vi "VIP_Post-Install Custom Action.vi"(10 "Variant":variant) -> (0 "error out":errorcluster)   [LabVIEW 2021]
uses:
  <vilib>/Utility/sysdir.llb/System Directory Type.ctl
  <userlib>/_OpenG.lib/lvzip/fileutil.llb/subVIs/FILE Rename (Path)__ogtk.vi
  <userlib>/_OpenG.lib/file/file.llb/openg_file.lvlib
  <userlib>/_OpenG.lib/file/file.llb/Convert File Extension (Path)__ogtk.vi
panel:
  # "POST INSTALL"
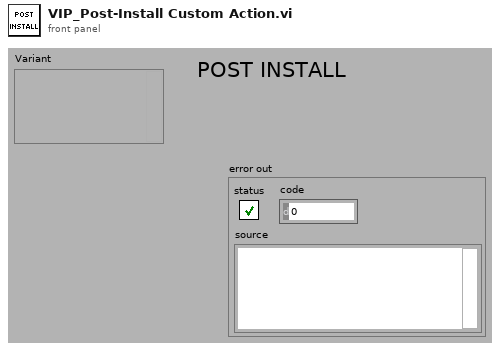
[diagram p1: front panel]
types:
  T1 = typedef "System Directory Type.ctl" = i32
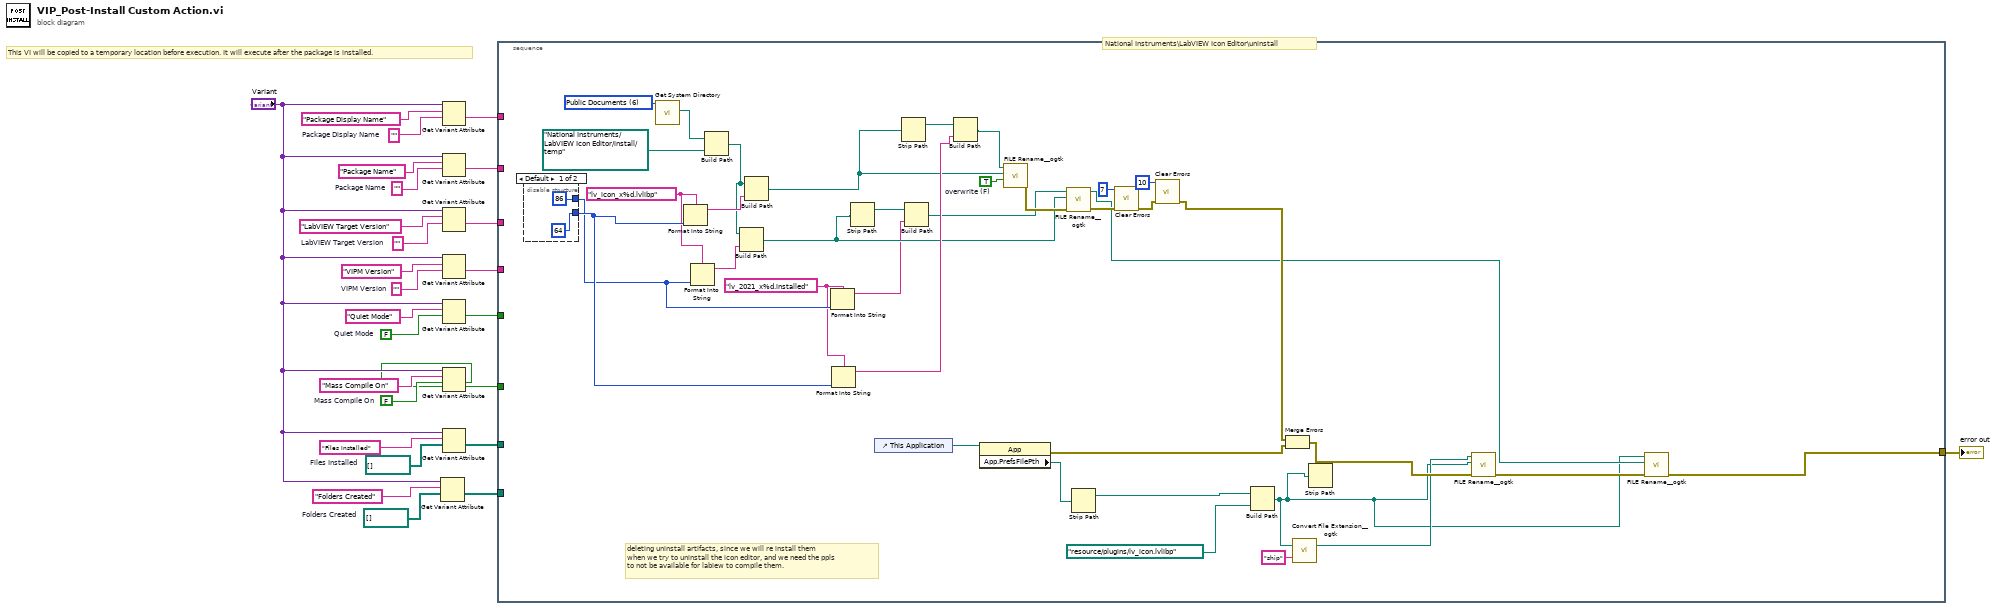
[diagram p0: block diagram]
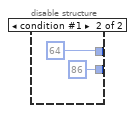
[diagram p2: hidden frame]
diagram:
  w10 = path[] []  # Folders Created
  w11 = path[] []  # Files Installed
  w15 = FALSE  # Mass Compile On
  w16 = ""  # Package Display Name
  w17 = FALSE  # Quiet Mode
  w20 = ""  # VIPM Version
  w22 = ""  # LabVIEW Target Version
  w24 = ""  # Package Name
  # "National Instruments\\LabVIEW Icon Editor\\uninstall"
  # "This VI will be copied to a temporary location before execution. It will execute after the package is installed."
  n1 = Get Variant Attribute(Variant="Variant", name="Folders Created", default value (empty Variant)=w10) -> (value=w2:path[])  [unwired: 1 in, 3 out]
  n2 = Get Variant Attribute(Variant="Variant", name="Package Display Name", default value (empty Variant)=w16) -> (value=w9:string)  [unwired: 1 in, 3 out]
  n3 = Get Variant Attribute(Variant="Variant", name="Package Name", default value (empty Variant)=w24) -> (value=w8:string)  [unwired: 1 in, 3 out]
  n4 = Get Variant Attribute(Variant="Variant", name="LabVIEW Target Version", default value (empty Variant)=w22) -> (value=w7:string)  [unwired: 1 in, 3 out]
  n5 = Get Variant Attribute(Variant="Variant", name="VIPM Version", default value (empty Variant)=w20) -> (value=w6:string)  [unwired: 1 in, 3 out]
  n6 = Get Variant Attribute(Variant="Variant", name="Quiet Mode", default value (empty Variant)=w17) -> (value=w3:bool)  [unwired: 1 in, 3 out]
  n7 = Get Variant Attribute(Variant="Variant", name="Mass Compile On", default value (empty Variant)=w15) -> (value=w5:bool)  [unwired: 1 in, 3 out]
  n8 = Get Variant Attribute(Variant="Variant", name="Files Installed", default value (empty Variant)=w11) -> (value=w4:path[])  [unwired: 1 in, 3 out]
  n9 = stacked-sequence {
    tunnel: [w28] -> w1
    tunnel: w9 -> [_]
    tunnel: w8 -> [_]
    tunnel: w7 -> [_]
    tunnel: w6 -> [_]
    tunnel: w5 -> [_]
    tunnel: w4 -> [_]
    tunnel: w3 -> [_]
    tunnel: w2 -> [_]
    frame #0 {
      w41 = "lv_2021_x%d.installed" ("format string")
      w58 = TRUE  # overwrite (F)
      w40 = "lv_icon_x%d.lvlibp" ("format string")
      w63 = T1 6 items=["User Home"=0, "User Desktop"=1, "User Documents"=2, "User Application Data"=3, "User Preferences"=4, "User Temporary"=5, "Public Documents"=6, "Public Application Data"=7, "Public Preferences"=8, "Public Cache"=13, "System Core Libraries"=9, "System Installed Libraries"=10, "Application Files"=11, "Boot Volume Root"=12] ("system directory type")
      # "deleting uninstall artifacts, since we will re install them\nwhen we try to uninstall the icon editor, and we need the ppls\nto not be available for labiew to compile them."
      n10 = disable-structure shown="Default" {
        disable-tunnel: [64 ("code") 86 ("code")] -> w57
        disable-tunnel: [86 ("code") 64 ("code")] -> w46
        frame condition #0 (active) {
        }
        frame condition #1 {
        }
      }
      n11 = call <vilib>:"Get System Directory.vi"("system directory type"=w63) -> ("system directory"=w35:path)  [unwired: 10 in]
      n12 = Format Into String(format string=w40, w57) -> (resulting string=w55:string)  [unwired: 2 in, 1 out]
      n13 = Format Into String(format string=w40, w46) -> (resulting string=w50:string)  [unwired: 2 in, 1 out]
      n14 = Build Path(base path=w35, name or relative path=path "National Instruments/LabVIEW Icon Editor/install/temp" ("source path")) -> (appended path=w51:path)
      n15 = Build Path(base path=w51, name or relative path=w50) -> (appended path=w47:path)
      n16 = Build Path(base path=w51, name or relative path=w55) -> (appended path=w36:path)
      n17 = Format Into String(format string=w41, w46) -> (resulting string=w45:string)  [unwired: 2 in, 1 out]
      n18 = Format Into String(format string=w41, w57) -> (resulting string=w53:string)  [unwired: 2 in, 1 out]
      n19 = Strip Path(path=w47) -> (stripped path=w48:path)  [unwired: 1 out]
      n20 = control-ref of="This Application"() -> (w62:refnum<vi>)
      n21 = Strip Path(path=w36) -> (stripped path=w54:path)  [unwired: 1 out]
      n22 = Build Path(base path=w48, name or relative path=w45) -> (appended path=w44:path)
      n23 = Build Path(base path=w54, name or relative path=w53) -> (appended path=w52:path)
      n24 = property class="App"(reference=w62) -> (error out=w59:errorcluster, "App.PrefsFilePth"=w60:path)  [unwired: 1 in, 1 out]
      n25 = call-poly <userlib>:"FILE Rename__ogtk.vi"("overwrite (F)"=w58, "source path"=w36, "target path"=w52) -> ("error out"=w49:errorcluster)  [unwired: 7 in, 1 out]
      n26 = call-poly <userlib>:"FILE Rename__ogtk.vi"("error in (no error)"=w49, "source path"=w47, "target path"=w44) -> ("error out"=w43:errorcluster, "dup target path"=w30:path)  [unwired: 7 in]
      n27 = Strip Path(path=w60) -> (stripped path=w33:path)  [unwired: 1 out]
      n28 = call <vilib>:"Clear Errors.vi"("error in (no error)"=w43, "specific error code to clear (0: all)"=7) -> ("error out"=w39:errorcluster)  [unwired: 4 in, 1 out]
      n29 = call <vilib>:"Clear Errors.vi"("error in (no error)"=w39, "specific error code to clear (0: all)"=10) -> ("error out"=w38:errorcluster)  [unwired: 4 in, 1 out]
      n30 = Build Path(base path=w33, name or relative path=path "resource/plugins/lv_icon.lvlibp") -> (appended path=w27:path)
      n31 = Merge Errors(w38, w59) -> (w32:errorcluster)
      n32 = call-poly <userlib>:"Convert File Extension__ogtk.vi"("new ending (none)"="ship", "file name"=w27) -> ("new filename"=w31:path)  [unwired: 1 out]
      n33 = Strip Path(path=w27) -> ()  [unwired: 2 out]
      n34 = call-poly <userlib>:"FILE Rename__ogtk.vi"("error in (no error)"=w32, "source path"=w27, "target path"=w31) -> ("error out"=w29:errorcluster)  [unwired: 7 in, 1 out]
      n35 = call-poly <userlib>:"FILE Rename__ogtk.vi"("error in (no error)"=w29, "source path"=w30, "target path"=w27) -> ("error out"=w28:errorcluster)  [unwired: 7 in, 1 out]
    }
  }
  "error out" <- w1
